vi "Background Loop Step.vi"(8 "error in (no error)":errorcluster, 10 "Action":T1, 11 "Red Pitaya Digitizer in":refnum<class "Red Pitaya Digitizer.lvclass">) -> (0 "error out":errorcluster, 1 "Next step delay":i32, 2 "Action out":T1, 3 "Red Pitaya Digitizer out":refnum<class "Red Pitaya Digitizer.lvclass">, 4 "Result":refnum<class "Acquired Result.lvclass">)   [LabVIEW 2024, in "Red Pitaya Digitizer.lvclass"]
uses:
  Red Pitaya Digitizer.lvclass
  LabActor/Worker/Worker Actor/Background Loop Action.ctl
  Instruments/Results/Acquired Result/Acquired Result.lvclass
  LabActor/Controllers/Process Controller/Request type.ctl
  <vilib>/Utility/error.llb/Error Cluster From Error Code.vi
  RP Core/RP Instrument/RP Instrument.lvclass
  <vilib>/ErrorRing/Error Ring.xnode
  Red Pitaya Digitizer.lvclass/Red Pitaya Digitizer.ctl
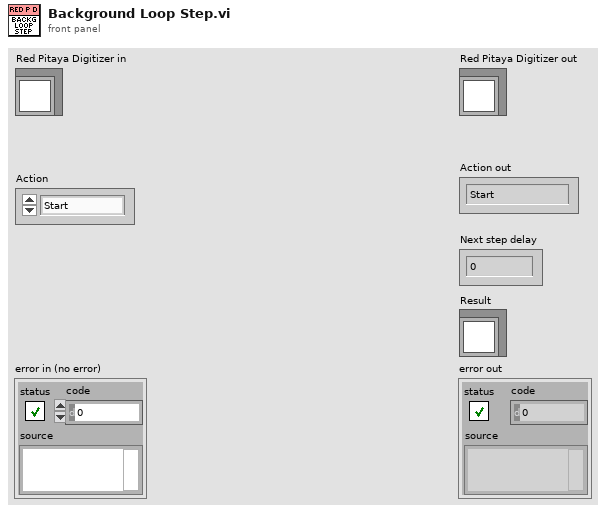
[diagram p1: front panel]
types:
  T1 = typedef "Background Loop Action.ctl" = enum16{"Start", "Continue", "Stop"}
  T2 = typedef "Request type.ctl" = enum16{"Process complete", "User command", "Auto-restart", "Error"}
  T3 = typedef "Lockin Digitizer Configuration.ctl" = cluster{"Post-trigger delay":dbl, "Post-trigger duration":dbl, "Rate":dbl, "Ranges":dbl[], "Re-name channels":string[], "Active channels":string, "External\nclock":bool, "Monitor time\nconstant":dbl, "Sync":bool, "Lock-in input channel phases":dbl[], "Output channels configuration":T4[]}
  T4 = typedef "Output Channel Configuration.ctl" = cluster{"Input channels":string, "Frequency":dbl, "Output amplitude":dbl, "Output channel number":i32}
  T5 = typedef "L-D Command Context.ctl" = enum16{"Re", "Switch", "Measure", "Arm"}
  T6 = map{i32, cluster{"Module":i32, "Local channel":i32}}
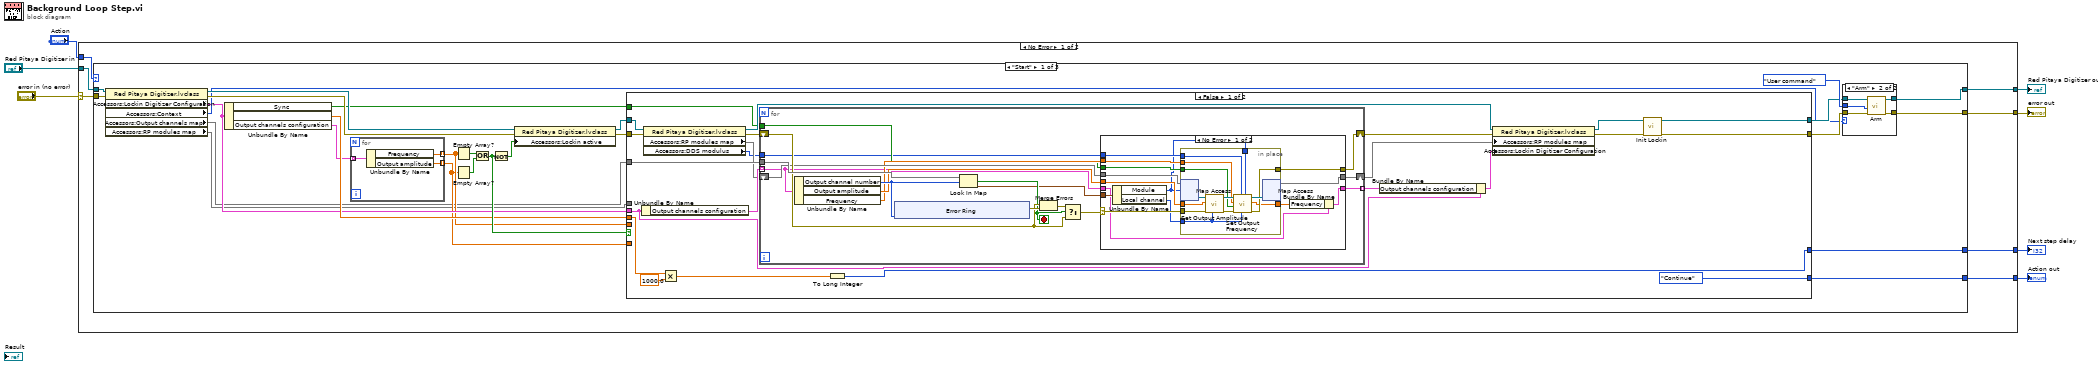
[diagram p0: block diagram]
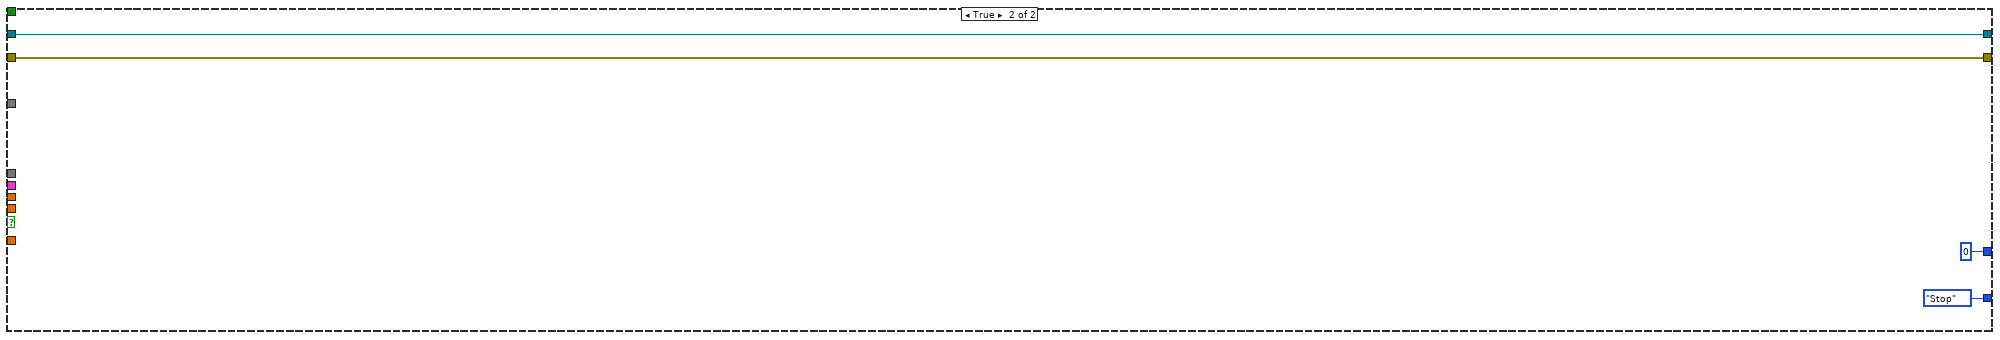
[diagram p4: hidden frame]
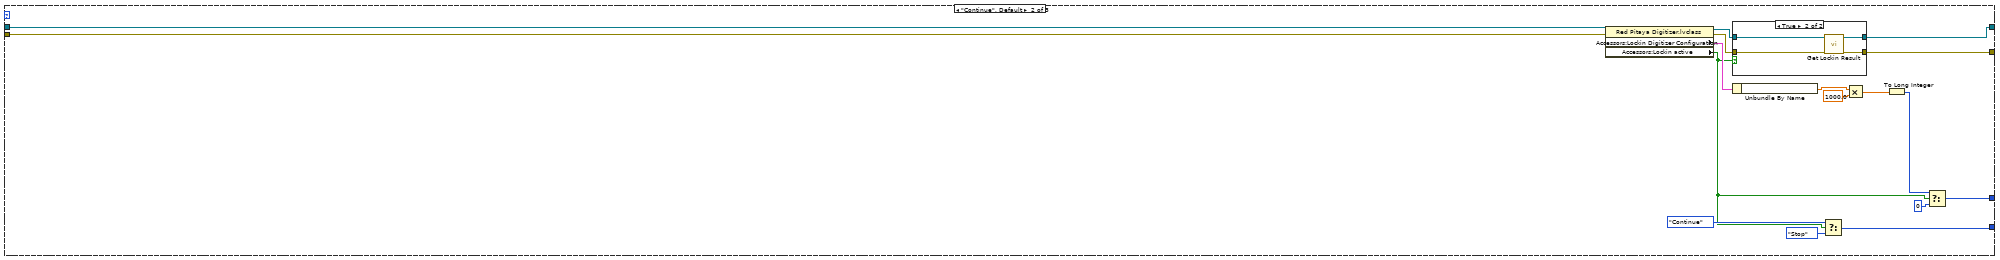
[diagram p5: hidden frame]
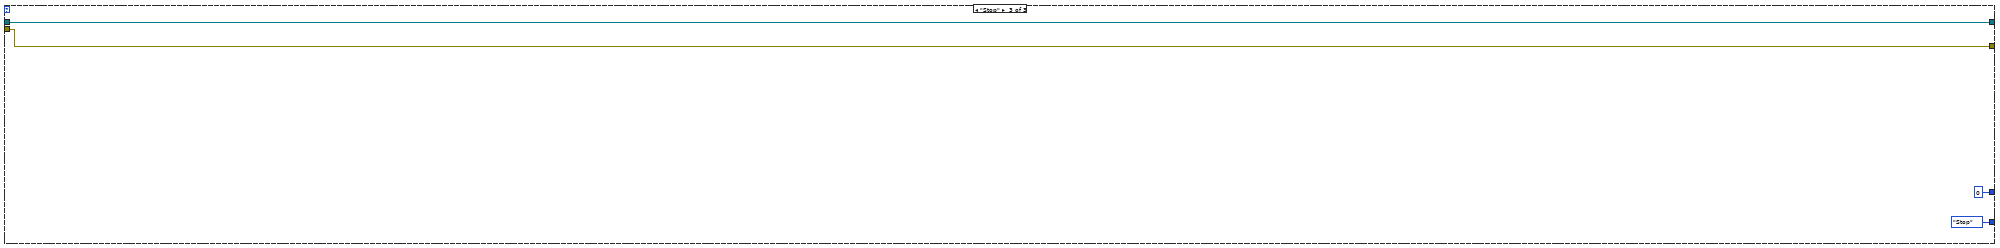
[diagram p7: hidden frame]
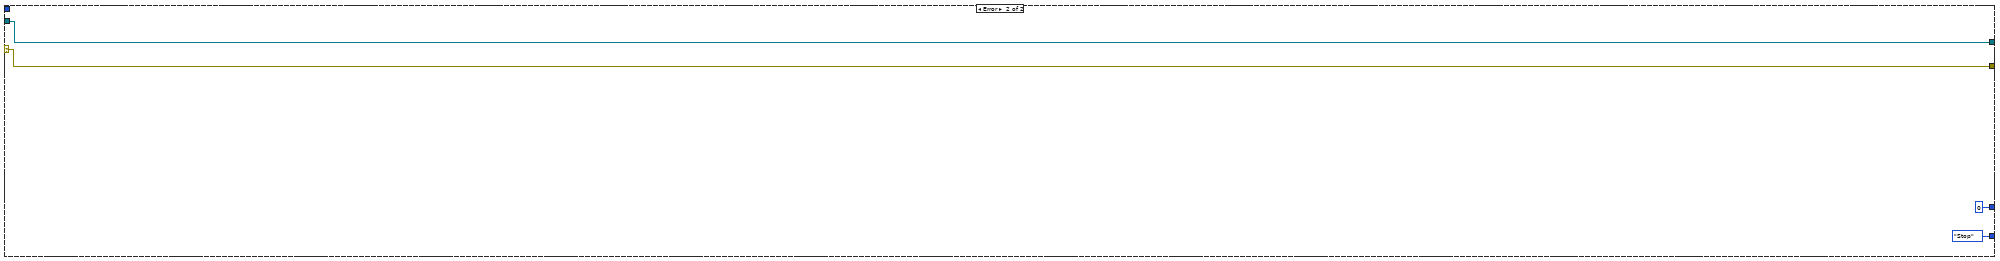
[diagram p8: hidden frame]
diagram:
  n1 = case shown="No Error" "error in (no error)" {
    selector: "error in (no error)" -> [w13 w161]
    tunnel: "Action" -> [w14 _]
    tunnel: "Red Pitaya Digitizer in" -> [w12 w162]
    tunnel: [w11 w162] -> w4
    tunnel: [w10 w161] -> w3
    tunnel: [w9 Background_Loop_Action."Stop" ("f")] -> w2
    tunnel: [w8 0 ("f")] -> w1
    frame No Error {
      n2 = case shown="\"Start\"" w14 {
        tunnel: w13 -> [w40 w137 w157]
        tunnel: w12 -> [w36 w138 w158]
        tunnel: [w39 w134 w158] -> w11
        tunnel: [w37 w132 w157] -> w10
        tunnel: [w25 w139 Background_Loop_Action."Stop" ("f")] -> w9
        tunnel: [w24 w143 0 ("f")] -> w8
        frame "Start" {
          n3 = property class="Red Pitaya Digitizer.lvclass"(reference=w36, error in=w40) -> (reference out=w29:refnum<class "Red Pitaya Digitizer.lvclass">, error out=w33:errorcluster, "Accessors:Lockin Digitizer Configuration"=w21:T3, "Accessors:Context"=w22:T5, "Accessors:Output channels map"=w16:T6, "Accessors:RP modules map "=w15:map{i32, refnum<class "RP Instrument.lvclass">})
          n4 = Unbundle By Name(w21) -> ("Sync"=w20:bool, "Monitor time\nconstant"=w23:dbl, "Output channels configuration"=w19:T4[])
          n5 = for {
            tunnel: w19 -> [w43] mode=indexing
            tunnel: [w42] -> w18 mode=indexing
            tunnel: [w41] -> w17 mode=indexing
            n6 = Unbundle By Name(w43) -> ("Frequency"=w42:dbl, "Output amplitude"=w41:dbl)
          }
          n7 = Empty Array?(array=w18) -> (empty?=w35:bool)
          n8 = Empty Array?(array=w17) -> (empty?=w34:bool)
          n9 = Or(x=w35, y=w34) -> (x .or. y?=w27:bool)
          n10 = Not(x=w27) -> (.not. x?=w26:bool)
          n11 = property class="Red Pitaya Digitizer.lvclass"(reference=w29, error in=w33, "Accessors:Lockin active"=w26) -> (reference out=w28:refnum<class "Red Pitaya Digitizer.lvclass">, error out=w30:errorcluster)
          n12 = case shown="False" w27 {
            tunnel: w18 -> [_ _]
            tunnel: w17 -> [_ _]
            tunnel: w30 -> [w58 w131]
            tunnel: [w64 w131] -> w32
            tunnel: w28 -> [w73 w130]
            tunnel: [w65 w130] -> w31
            tunnel: [Background_Loop_Action."Continue" ("Action out") Background_Loop_Action."Stop" ("Action out")] -> w25
            tunnel: [w67 0 ("Next step delay")] -> w24
            tunnel: w23 -> [w70 _]
            tunnel: w20 -> [w57 _]
            tunnel: w21 -> [w61 _]
            tunnel: w16 -> [w59 _]
            tunnel: w15 -> [_ _]
            frame False {
              n13 = Unbundle By Name(w61) -> ("Output channels configuration"=w60:T4[])
              n14 = property class="Red Pitaya Digitizer.lvclass"(reference=w73, error in=w58) -> (reference out=w72:refnum<class "Red Pitaya Digitizer.lvclass">, error out=w52:errorcluster, "Accessors:RP modules map "=w54:map{i32, refnum<class "RP Instrument.lvclass">}, "Accessors:DDS modulus"=w51:i64)
              n15 = Multiply(x=w70, y=1000.0) -> (x*y=w69:dbl)
              n16 = for {
                tunnel: w60 -> [w76] mode=indexing
                tunnel: w59 -> [w90]
                shift-right: [w78] -> w53
                shift-left: w52 -> [w87]
                tunnel: w57 -> [w79]
                shift-right: [w77] -> w56
                shift-left: w54 -> [w82]
                tunnel: [w75] -> w55 mode=indexing
                tunnel: w51 -> [w74]
                stop <- w86 stop-if-true
                n17 = Unbundle By Name(w76) -> ("Output channel number"=w85:i32, "Output amplitude"=w81:dbl, "Frequency"=w80:dbl)
                n18 = xnode "Error Ring"("parameter 0"=w85) -> ("error out"=w88:errorcluster)
                n19 = Look In Map(map=w90, key=w85) -> (key not found?=w86:bool, value=w83:cluster{"Module":i32, "Local channel":i32})  [unwired: 1 in]
                n20 = Merge Errors(w87, w88) -> (w89:errorcluster)
                n21 = Select(t=w89, s=w86, f=w87) -> (s? t:f=w84:errorcluster)
                n22 = case shown="No Error" w84 {
                  selector: w84 -> [w102 w120]
                  tunnel: w83 -> [w104 _]
                  tunnel: w82 -> [w103 w119]
                  tunnel: w81 -> [w100 _]
                  tunnel: w80 -> [w99 _]
                  tunnel: w79 -> [w98 _]
                  tunnel: [w97 w120] -> w78
                  tunnel: [w96 w119] -> w77
                  tunnel: w76 -> [w95 w118]
                  tunnel: [w93 w118] -> w75
                  tunnel: w74 -> [w92 _]
                  frame No Error {
                    n23 = Unbundle By Name(w104) -> ("Module"=w91:i32, "Local channel"=w101:i32)
                    n24 = in-place {
                      in-place-border: w102 -> [w113]
                      in-place-border: w101 -> [w112]
                      in-place-border: w100 -> [w111]
                      in-place-border: w99 -> [w110]
                      in-place-border: w98 -> [w109]
                      in-place-border: [w108] -> w97
                      in-place-border: [w107] -> w94
                      in-place-border: w92 -> [w106]
                      in-place-border: w91 -> [w105]
                      n25 = in-place-map #1(w103, w91) -> (w115:refnum<class "RP Instrument.lvclass">)  [unwired: 1 in, 1 out]
                      n26 = call-dynamic "Set Output Amplitude.vi"("Output channel"=w112, "error in (no error)"=w113, "Output amplitude"=w111, "RP Instrument in"=w115) -> ("error out"=w116:errorcluster, "RP Instrument out"=w117:refnum<class "RP Instrument.lvclass">)  [unwired: 6 in]
                      n27 = call-dynamic "Set Output Frequency.vi"("Module"=w105, "Output channel"=w112, "Original DDS modulus"=w106, "error in (no error)"=w116, "Synchronous"=w109, "Frequency"=w110, "RP Instrument in"=w117) -> ("error out"=w108:errorcluster, "Actual frequency"=w107:dbl, "RP Instrument out"=w114:refnum<class "RP Instrument.lvclass">)  [unwired: 2 in]
                      n28 = in-place-map #1(w114) -> (w96:map{i32, refnum<class "RP Instrument.lvclass">})  [unwired: 1 in, 2 out]
                    }
                    n29 = Bundle By Name(cluster=w95, "Frequency"=w94) -> (w93:T4)
                  }
                  frame Error {
                  }
                }
              }
              n30 = To Long Integer(number=w69) -> (32bit integer=w67:i32)
              n31 = Bundle By Name(cluster=w61, "Output channels configuration"=w55) -> (w62:T3)
              n32 = property class="Red Pitaya Digitizer.lvclass"(reference=w72, error in=w53, "Accessors:RP modules map "=w56, "Accessors:Lockin Digitizer Configuration"=w62) -> (reference out=w66:refnum<class "Red Pitaya Digitizer.lvclass">, error out=w63:errorcluster)
              n33 = call-dynamic "Init Lockin.vi"("error in (no error)"=w63, "Red Pitaya Digitizer in"=w66) -> ("error out"=w64:errorcluster, "Red Pitaya Digitizer out"=w65:refnum<class "Red Pitaya Digitizer.lvclass">)  [unwired: 8 in]
            }
            frame True {
            }
          }
          n34 = case shown="\"Arm\"" w22 {
            tunnel: [w45 w50] -> w39
            tunnel: Request_type."User command" ("Request type") -> [_ w49]
            tunnel: [w44 w48] -> w37
            tunnel: w32 -> [w44 w47]
            tunnel: w31 -> [w45 w46]
            frame "Re", Default {
            }
            frame "Arm" {
              n35 = call-dynamic "Arm.vi"("error in (no error)"=w47, "Request type"=w49, "Pulse Driver in"=w46) -> ("error out"=w48:errorcluster, "Pulse Driver out"=w50:refnum<class "Red Pitaya Digitizer.lvclass">)  [unwired: 6 in, 1 out]
            }
          }
        }
        frame "Continue", Default {
          n36 = property class="Red Pitaya Digitizer.lvclass"(reference=w138, error in=w137) -> (reference out=w135:refnum<class "Red Pitaya Digitizer.lvclass">, error out=w133:errorcluster, "Accessors:Lockin Digitizer Configuration"=w148:T3, "Accessors:Lockin active"=w136:bool)
          n37 = case shown="True" w136 {
            tunnel: w135 -> [w150 w154]
            tunnel: [w150 w153] -> w134
            tunnel: w133 -> [w149 w152]
            tunnel: [w149 w151] -> w132
            frame False {
            }
            frame True {
              n38 = call-dynamic "Get Lockin Result.vi"("error in (no error)"=w152, "Red Pitaya Digitizer in"=w154) -> ("error out"=w151:errorcluster, "Red Pitaya Digitizer out"=w153:refnum<class "Red Pitaya Digitizer.lvclass">)  [unwired: 6 in, 2 out]
            }
          }
          n39 = Unbundle By Name(w148) -> ("Monitor time\nconstant"=w145:dbl)
          n40 = Select(t=Background_Loop_Action."Continue" ("Action out"), s=w136, f=Background_Loop_Action."Stop") -> (s? t:f=w139:T1)
          n41 = Multiply(x=w145, y=1000.0) -> (x*y=w147:dbl)
          n42 = To Long Integer(number=w147) -> (32bit integer=w144:i32)
          n43 = Select(t=w144, s=w136, f=0) -> (s? t:f=w143:i32)
        }
        frame "Stop" {
        }
      }
    }
    frame Error {
    }
  }
  "error out" <- w3
  "Red Pitaya Digitizer out" <- w4
  "Next step delay" <- w1
  "Action out" <- w2
